vi "ReadText_Subvi.vi"(11 "index":i32=1) -> (2 "Position(mm)":i32=20, 3 "size(s)":i32=9)   [LabVIEW 2018]
panel:
  out "EOF?":bool
  in  "delimiter (Tab)":string="\t"
  in  "type (empty)":string[][](array[string])
  in  "transpose (no:F)":bool
  in  "format (%.3f)":string="%.3f"
  out "all rows":string[][](array[string])=[["0"], ["20"], ["1"], ["20"], ["2"], ["20"], ["3"], ["0"], ["-1"]]
  in  "number of rows (all:-1)":i32=-1
  out "mark after read (chars.)":i32=29
  in  "max characters/row  (no limit:0)":i32
  in  "start of read offset (chars.:0)":i32
  in  "file path (dialog if empty)":path=path "C:/Users/Academia Sinica/Desktop/AutoSampler _GB/AutoSampler.txt"
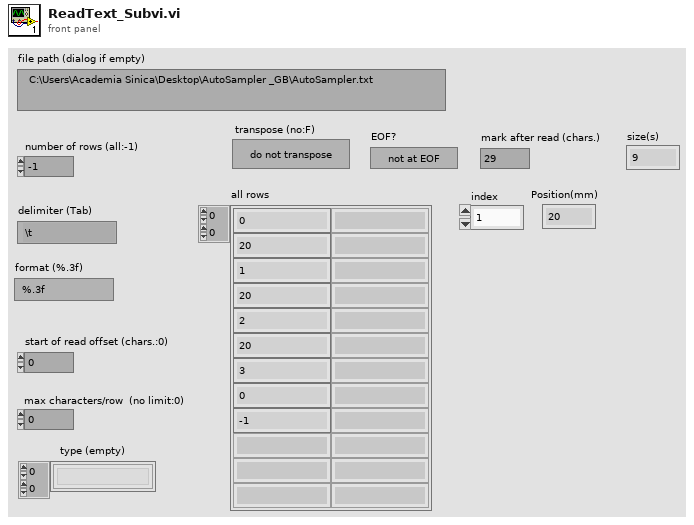
[diagram p1: front panel]
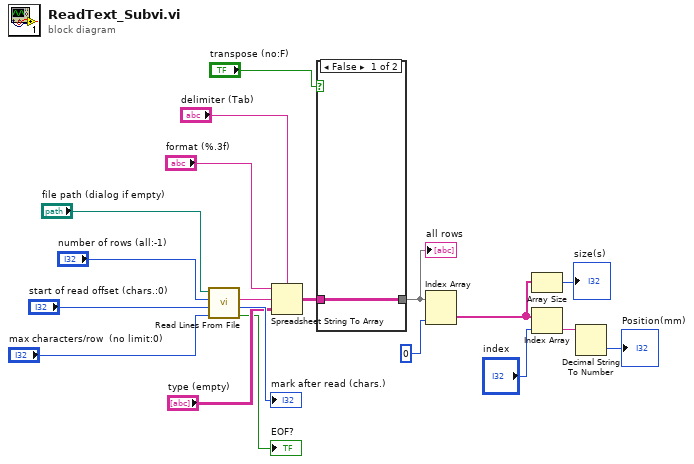
[diagram p0: block diagram]
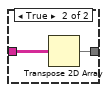
[diagram p2: hidden frame]
diagram:
  n1 = call <vilib>:"Read Lines From File.vi"("file path (dialog if empty)"="file path (dialog if empty)", "number of lines (all:-1)"="number of rows (all:-1)", "start of read offset (chars.:0)"="start of read offset (chars.:0)", "[max characters per line]  (no limit:0)"="max characters/row  (no limit:0)") -> ("line string"=w15:string, "mark after read (chars.)"=→"mark after read (chars.)":i32, "EOF?"=→"EOF?":bool)  [unwired: 2 in, 1 out]
  n2 = Spreadsheet String To Array(delimiter (Tab)="delimiter (Tab)", format string="format (%.3f)", spreadsheet string=w15, array type (2D Dbl)="type (empty)") -> (array=w13:string[][])
  n3 = case shown="False" "transpose (no:F)" {
    tunnel: [w20 w22] -> w7
    tunnel: w13 -> [w20 w21]
    frame False {
    }
    frame True {
      n4 = Transpose 2D Array(2D array=w21) -> (transposed array=w22:string[][])
    }
  }
  "all rows" <- w7
  n5 = Index Array "Index Array"(array=w7, index (col)=0) -> (element=w5:string[])  [unwired: 1 in]
  n6 = Array Size(array=w5) -> (size(s)=→"size(s)":i32)
  n7 = Index Array(array=w5, index="index") -> (element=w3:string)
  n8 = Decimal String To Number(string=w3) -> (number=→"Position(mm)":i32)  [unwired: 2 in, 1 out]
